vi "CPP-BLNormaliseToZref.vi"() -> (0 "New Values In":string[][](array[string]), 1 "New Chs In":string[](array[string]))   [LabVIEW 2013]
uses:
  Results_plotter_Global.vi
panel:
  in  "Zref":dbl=1000.0
  # "This VI receives \"classic\" transposed plots of U/Uref vs Z, and linearly interpolates to find a velocity at a given height.\nFor use when re-normalising profiles about a height other than their original reference.\nTry a test run first and set Zref as required before processing a batch of profiles!"
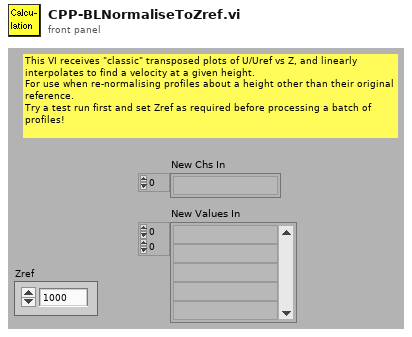
[diagram p1: front panel]
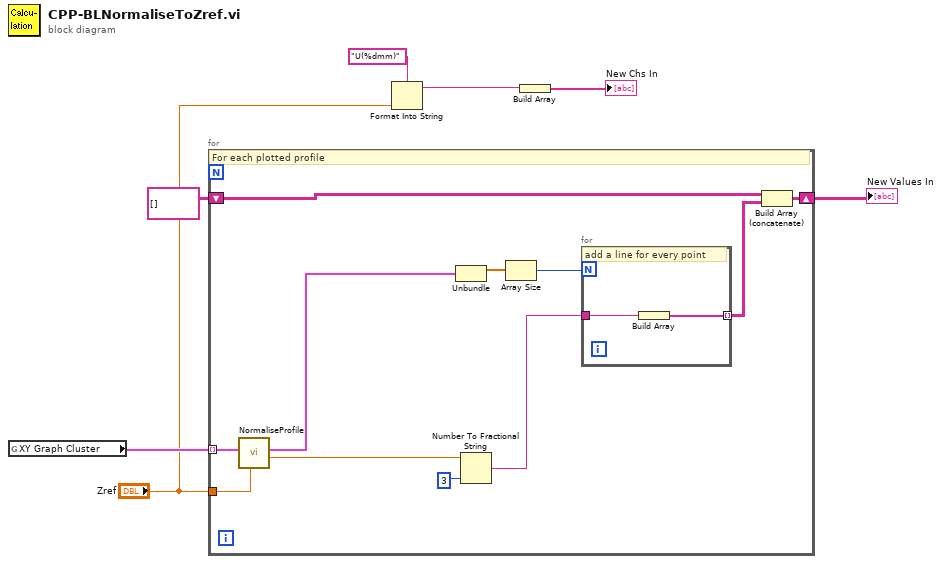
[diagram p0: block diagram]
diagram:
  n1 = global read "Results_plotter_Global.vi" "XY Graph Cluster"() -> (w6:cluster{dbl[], dbl[]}[])
  n2 = for {
    tunnel: "Zref" -> [w9]
    tunnel: w6 -> [w11] mode=indexing
    shift-right: [w16] -> w4
    shift-left: string[][] [] -> [w15]
    # "For each plotted profile"
    n3 = call "NormaliseProfile.vi"("Zref"=w9, "zUClusterIn"=w11) -> ("U(Zref)"=w8:dbl, "zUClusterNormalised"=w10:cluster{dbl[], dbl[]})  [unwired: 8 in]
    n4 = Unbundle(w10) -> (w13:dbl[])  [unwired: 1 out]
    n5 = Number To Fractional String(number=w8, precision (6)=i16 3) -> (F-format string=w17:string)  [unwired: 2 in]
    n6 = Array Size(array=w13) -> (size(s)=w14:i32)
    n7 = for {
      N: w14 -> [_]
      tunnel: w17 -> [w20]
      tunnel: [w19] -> w12 mode=indexing
      # "add a line for every point"
      n8 = Build Array(w20) -> (w19:string[])
    }
    n9 = Build Array (concatenate)(w15, w12) -> (w16:string[][])
  }
  "New Values In" <- w4
  n10 = Format Into String(format string="U(%dmm)", "Zref") -> (resulting string=w2:string)  [unwired: 2 in, 1 out]
  n11 = Build Array(w2) -> (→"New Chs In":string[])
